vi "Templating-Root.vi"(8 "error in (no error)":errorcluster) -> (0 "error out":errorcluster, 3 "Template-Root":path)   [LabVIEW 2018, in "Scripting.lvlib"]
uses:
  Scripting.lvlib
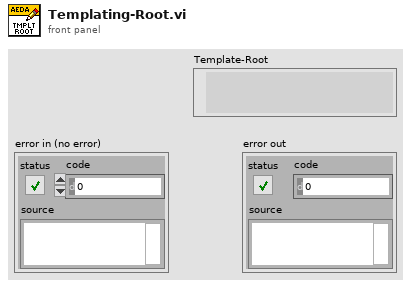
[diagram p1: front panel]
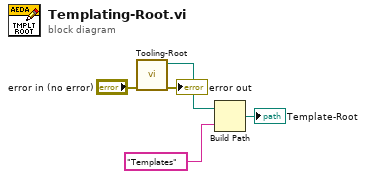
[diagram p0: block diagram]
diagram:
  n1 = call "Tooling-Root.vi"("error in (no error)"="error in (no error)") -> ("error out"=→"error out":errorcluster, "Root"=w5:path)  [unwired: 9 in]
  n2 = Build Path(base path=w5, name or relative path="Templates") -> (appended path=→"Template-Root":path)
